vi "New Image (RGBA).vi"(3 "Error":string, 4 "Height":i16, 5 "Width":i16) -> (0 "Error":string, 2 "VVIS Image":T1={"Image ID"=0, "Channel ID"=-1})   [LabVIEW 2011, in "labvvis.lvlib"]
doc: "Creates a new RGBA image. Each channel within this image is 8-bit. Please delete this image when it is no longer required.\n\nThe initial value of pixels within the newly created image is undefined."
uses:
  <userlib>/labvvis/labvvis.lvlib
  <userlib>/labvvis/VVIS Image.ctl
  labvvis.framework
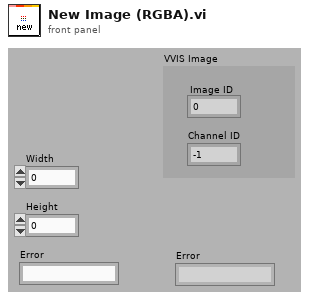
[diagram p1: front panel]
types:
  T1 = typedef "labvvis.lvlib/VVIS Image.ctl" = cluster{"Image ID":i16, "Channel ID":i16}
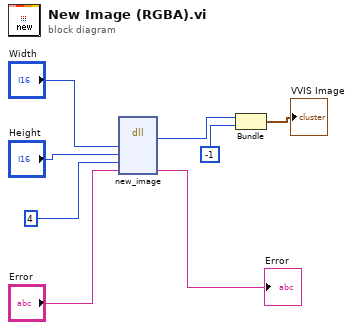
[diagram p0: block diagram]
diagram:
  n1 = dll-call lib="labvvis.framework" fn="new_image"("width"="Width", "height"="Height", "channel_count"=i16 4, "error"="Error") -> (w8:i16, "error"=→"Error":string)  [unwired: 6 in, 2 out]
  n2 = Bundle(w8, -1) -> (→"VVIS Image":cluster{i16, i32})  [unwired: 1 in]
